vi "Set Arm State.vi"(8 "error in":errorcluster, 9 "PotDevRef":T12={"DevStatus"={"status"=FALSE, "code"=0, "source"=""}, "Controller"=enum."Controller 1", "Analog Channel"=enum."AI 2", "Invert Output"=FALSE}, 10 "MotorControlDevRef":T3={"DeviceStatus"={"status"=FALSE, "code"=0, "source"=""}, "Type"=enum."CANTalonSRX", "PWM"={"Controller"=enum."Controller 1", "PWM Channel"=enum."PWM 1", "DeadBand"={"Name"="", "maxPositivePwm"=0, "minPositivePwm"=0, "centerPwm"=0, "maxNegativePwm"=0, "minNegativePwm"=0, "angularRange"=0}}, "CAN"={"Device Number"=2, "Control Mode"=enum."Percent VBus", "Semaphore"=refnum, "Max Vout"=12.0, "TalonSRX Control Mode"=enum."Percent VBus"}, "Invert"=TRUE, "TransformRef"=refnum, "InvTransformRef"=refnum}, 11 "State":T2) -> (0 "error out":errorcluster, 1 "Good enough?":bool=TRUE)   [LabVIEW 2014]
doc: "Actuate the arm motors using a PID loop based on the next state."
uses:
  Arm State.ctl
  <vilib>/Rock Robotics/WPI/Potentiometer/WPI_PotentiometerDevRef.ctl
  <vilib>/Rock Robotics/SystemInterfaces/Typedef/FPGA_TypedefAnalogModule.ctl
  <vilib>/Rock Robotics/SystemInterfaces/AI/FPGA_AIChannel.ctl
  <vilib>/Rock Robotics/WPI/MotorControl/WPI_MotorControlDeviceRef.ctl
  <vilib>/Rock Robotics/WPI/MotorControl/WPI_MotorControlType.ctl
  <vilib>/Rock Robotics/SystemInterfaces/Typedef/FPGA_TypedefDigitalModule.ctl
  <vilib>/Rock Robotics/SystemInterfaces/DIO/FPGA_DIOPWMChannel.ctl
  <vilib>/Rock Robotics/WPI/PWM/WPI_PWMDeadband.ctl
  <vilib>/Rock Robotics/WPI/CAN/Jaguar/SubVIs/WPI_CANJaguar_ControlMode.ctl
  <vilib>/Rock Robotics/WPI/CAN/TalonSRX/WPI_CANTalonSRX_APIControlMode.ctl
  <vilib>/Rock Robotics/WPI/PWM/WPI_PWMTransform_ConPane.ctl
  Arm Angle Control Mode.ctl
  <vilib>/Rock Robotics/WPI/DriverStation/WPI_DriverStationRobotMode2.ctl
  <vilib>/Rock Robotics/Network Tables/SD Read Boolean.vi
  Robot Global Data.vi
  <vilib>/addons/control/pid/pid.llb/PID (DBL).vi
  <vilib>/Rock Robotics/Network Tables/SD Write Number.vi
  <vilib>/addons/control/pid/NI_PID_pid.lvlib
panel:
  in  "Tolerance":dbl=0.05 format="%#_13g"
  in  "PID?":bool=TRUE
  in  "Formula":i32=2
  in  "Tab Control":T1(tab)=enum."PID"
  in  "Vertical Setpoint":dbl=0.516 format="%#_13g"
  in  "output range":cluster{"output high":dbl, "output low":dbl}={"output high"=1.0, "output low"=-1.0}
  in  "PID gains":T15={"proportional gain (Kc)"=5.0, "integral time (Ti, min)"=0.0, "derivative time (Td, min)"=0.0} {"proportional gain (Kc)" min=0.0 max=1000.0 step=0.01; "integral time (Ti, min)" min=0.0 max=1000.0 step=0.0001; "derivative time (Td, min)" min=0.0 max=10000.0 step=0.001}
  in  "Lower Setpoint":dbl=0.088 format="%#_13g"
  in  "Raise Setpoint":dbl=0.252 format="%#_13g"
  in  "Level Setpoint":dbl=0.148 format="%#_13g"
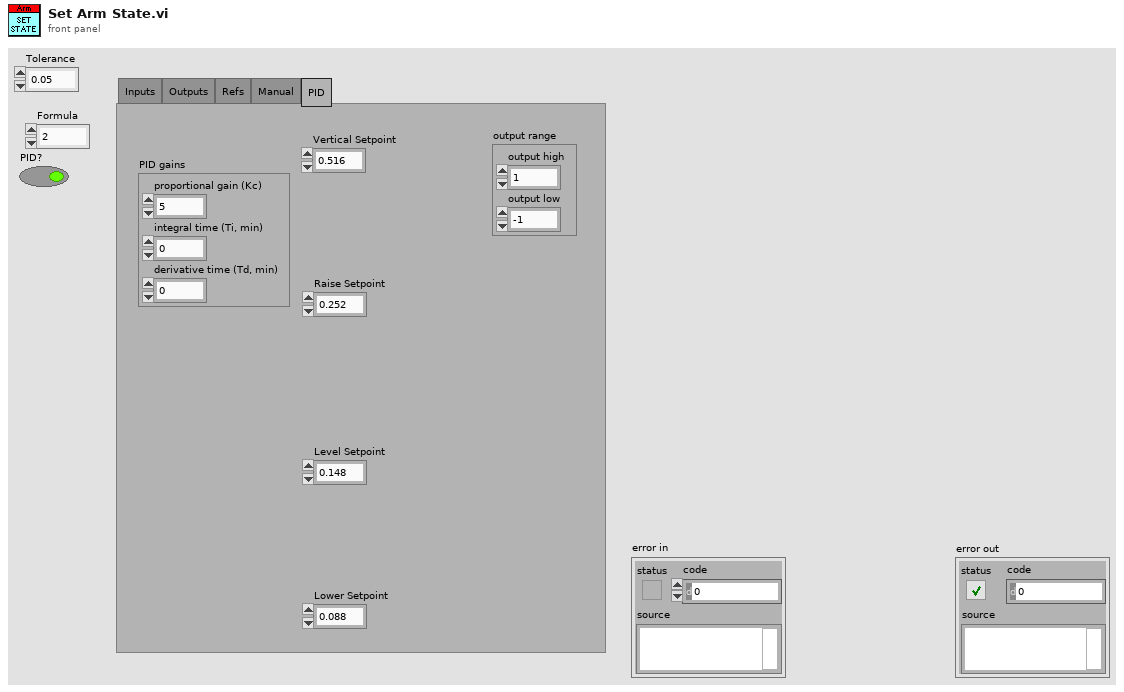
[diagram p1: front panel]
types:
  T1 = enum32{"Inputs", "Outputs", "Refs", "Manual", "PID"}
  T2 = typedef "Arm State.ctl" = enum16{"Ground", "Level", "Feeder", "Vertical"}
  T3 = typedef "WPI_MotorControlDeviceRef.ctl" = cluster{"DeviceStatus":errorcluster, "Type":T4, "PWM":cluster{"Controller":T5, "PWM Channel":T6, "DeadBand":T7}, "CAN":cluster{"Device Number":u8, "Control Mode":T8, "Semaphore":T9, "Max Vout":dbl, "TalonSRX Control Mode":T10}, "Invert":bool, "TransformRef":T11, "InvTransformRef":T11}
  T4 = typedef "WPI_MotorControlType.ctl" = enum16{"PWM", "CAN", "CANTalonSRX"}
  T5 = typedef "FPGA_TypedefDigitalModule.ctl" = enum16{"Controller 1"}
  T6 = typedef "FPGA_DIOPWMChannel.ctl" = enum8{"PWM 0", "PWM 1", "PWM 2", "PWM 3", "PWM 4", "PWM 5", "PWM 6", "PWM 7", "PWM 8", "PWM 9", "PWM MXP 0", "PWM MXP 1", "PWM MXP 2", "PWM MXP 3", "PWM MXP 4", "PWM MXP 5", "PWM MXP 6", "PWM MXP 7", "PWM MXP 8", "PWM MXP 9", "Invalid"}
  T7 = typedef "WPI_PWMDeadband.ctl" = cluster{"Name":string, "maxPositivePwm":i32, "minPositivePwm":i32, "centerPwm":i32, "maxNegativePwm":i32, "minNegativePwm":i32, "angularRange":u16}
  T8 = typedef "WPI_CANJaguar_ControlMode.ctl" = enum8{"Percent VBus", "Current", "Speed", "Position", "Voltage"}
  T9 = typedef "Semaphore RefNum" = refnum<k1>
  T10 = typedef "WPI_CANTalonSRX_APIControlMode.ctl" = enum8{"Percent VBus", "Speed", "Position", "Slave", "Unchanged / Invalid"}
  T11 = typedef "WPI_PWMTransform_ConPane.ctl" = refnum<vi>
  T12 = typedef "WPI_PotentiometerDevRef.ctl" = cluster{"DevStatus":errorcluster, "Controller":T13, "Analog Channel":T14, "Invert Output":bool}
  T13 = typedef "FPGA_TypedefAnalogModule.ctl" = enum16{"Controller 1"}
  T14 = typedef "FPGA_AIChannel.ctl" = enum8{"AI 0", "AI 1", "AI 2", "AI 3", "AI MXP 0", "AI MXP 1", "AI MXP 2", "AI MXP 3", "Invalid"}
  T15 = cluster{"proportional gain (Kc)":dbl, "integral time (Ti, min)":dbl, "derivative time (Td, min)":dbl}
  T16 = typedef "Arm Angle Control Mode.ctl" = enum16{"PID", "PID to Manual", "Manual"}
  T17 = typedef "WPI_DriverStationRobotMode2.ctl" = enum16{"Autonomous Disabled", "Autonomous Enabled", "Teleop Disabled", "Teleop Enabled", "Disconnected", "Finish", "Test Disabled", "Test Enabled", "Emergency Stopped"}
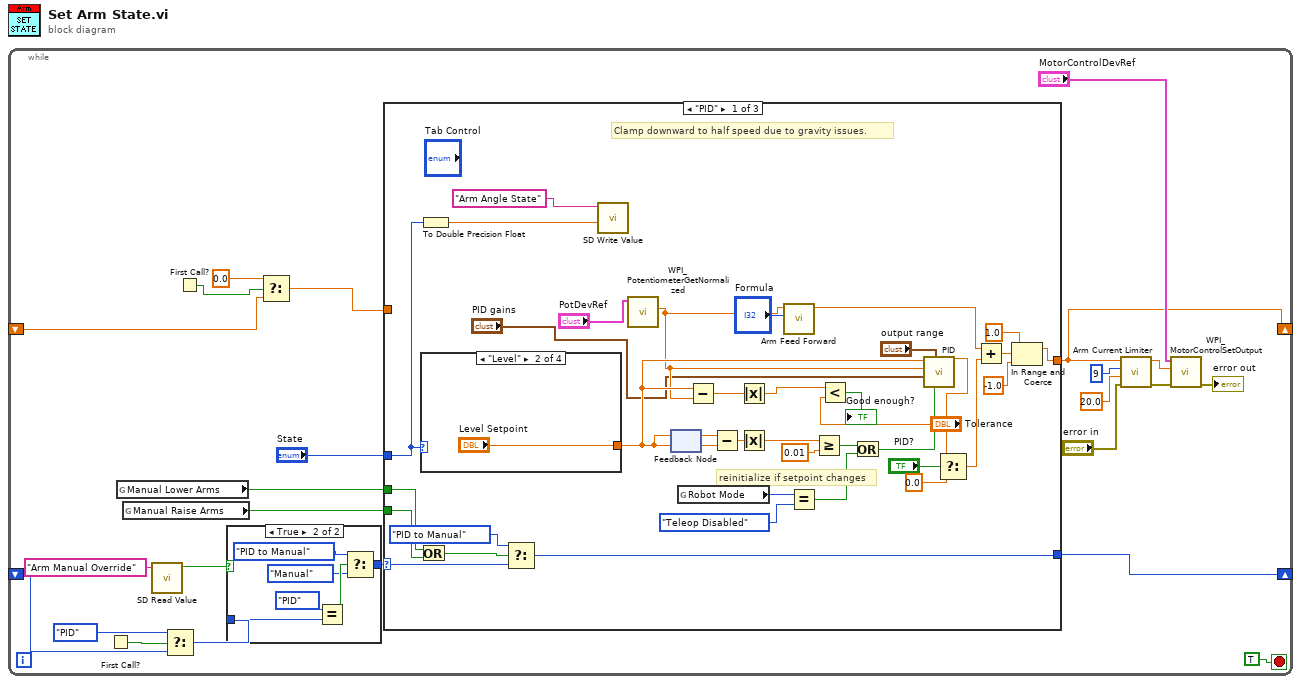
[diagram p0: block diagram]
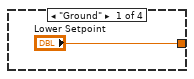
[diagram p3: hidden frame]
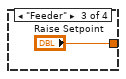
[diagram p4: hidden frame]
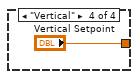
[diagram p5: hidden frame]
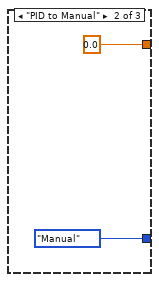
[diagram p6: hidden frame]
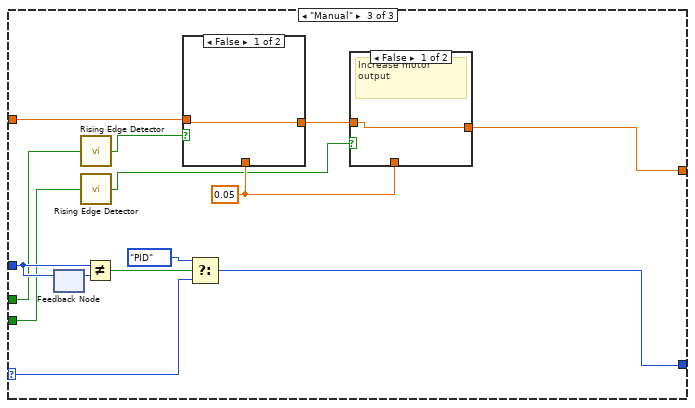
[diagram p7: hidden frame]
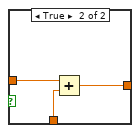
[diagram p8: hidden frame]
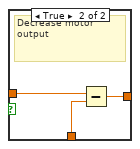
[diagram p9: hidden frame]
diagram:
  n1 = while {
    shift-right: [w23] -> _
    shift-left: _ -> [w18]
    shift-right: [w9] -> _
    shift-left: _ -> [w7]
    stop <- TRUE stop-if-true
    n2 = First Call?() -> (First Call?: T/F=w20:bool)
    n3 = global read "Robot Global Data.vi" "Manual Lower Arms"() -> (w22:bool)
    n4 = global read "Robot Global Data.vi" "Manual Raise Arms"() -> (w24:bool)
    n5 = call-poly <vilib>:"SD Read Value.vi"("Name"="Arm Manual Override") -> ("Boolean"=w3:bool)  [unwired: 8 in, 2 out]
    n6 = Select(t=Arm_Angle_Control_Mode."PID", s=w20, f=w18) -> (s? t:f=w2:T16)
    n7 = First Call?() -> (First Call?: T/F=w5:bool)
    n8 = case shown="True" w3 {
      tunnel: w2 -> [w25 w31]
      tunnel: [w25 w29] -> w1
      frame False {
      }
      frame True {
        n9 = Equal?(x=Arm_Angle_Control_Mode."PID", y=w31) -> (x = y?=w28:bool)
        n10 = Select(t=Arm_Angle_Control_Mode."PID to Manual", s=w28, f=Arm_Angle_Control_Mode."Manual") -> (s? t:f=w29:T16)
      }
    }
    n11 = Select(t=0.0, s=w5, f=w7) -> (s? t:f=w4:dbl)
    n12 = case shown="\"PID\"" w1 {
      selector: w1 -> [w65 _ w84]
      tunnel: "State" -> [w66 _ w85]
      tunnel: [w32 0.0 ("t") w80] -> w9
      tunnel: w22 -> [w67 _ w83]
      tunnel: w24 -> [w68 _ w82]
      tunnel: [w62 Arm_Angle_Control_Mode."Manual" w88] -> w23
      tunnel: w4 -> [_ _ w81]
      frame "PID" {
        # "Clamp downward to half speed due to gravity issues."
        # "reinitialize if setpoint changes"
        n13 = Or(x=w67, y=w68) -> (x .or. y?=w61:bool)
        n14 = To Double Precision Float(number=w66) -> (double precision float=w64:dbl)
        n15 = case shown="\"Level\"" w66 {
          tunnel: ["Lower Setpoint" "Level Setpoint" "Raise Setpoint" "Vertical Setpoint"] -> w45
          frame "Ground" {
          }
          frame "Level" {
          }
          frame "Feeder" {
          }
          frame "Vertical" {
          }
        }
        n16 = Select(t=Arm_Angle_Control_Mode."PID to Manual", s=w61, f=w65) -> (s? t:f=w62:T16)
        n17 = call-poly <vilib>:"SD Write Value.vi"("Numeric"=w64, "Name"="Arm Angle State") -> ()  [unwired: 8 in, 2 out]
        n18 = call <vilib>:"WPI_PotentiometerGetNormalized.vi"("PotDevRef"="PotDevRef") -> ("Normalized Value"=w43:dbl)  [unwired: 8 in, 2 out]
        n19 = feedback #1() -> (w44:dbl)  [unwired: 1 in]
        n20 = feedback-in #1(w45) -> ()
        n21 = global read "Robot Global Data.vi" "Robot Mode"() -> (w52:T17)
        n22 = Subtract(x=w45, y=w43) -> (x-y=w50:dbl)
        n23 = Subtract(x=w44, y=w45) -> (x-y=w56:dbl)
        n24 = Absolute Value(x=w50) -> (abs(x)=w49:dbl)
        n25 = Absolute Value(x=w56) -> (abs(x)=w57:dbl)
        n26 = call "Arm Feed Forward.vi"("Numeric"="Formula", "Arm Position"=w43) -> ("Feed Forward"=w42:dbl)  [unwired: 9 in]
        n27 = Equal?(x=w52, y=WPI_DriverStationRobotMode2."Teleop Disabled") -> (x = y?=w54:bool)
        n28 = Greater Or Equal?(x=w57, y=0.01) -> (x >= y?=w58:bool)
        n29 = Less?(x=w49, y="Tolerance") -> (x < y?=→"Good enough?":bool)
        n30 = Or(x=w58, y=w54) -> (x .or. y?=w59:bool)
        n31 = call-poly <vilib>:"PID.vi"("reinitialize? (F)"=w59, "output range"="output range", "PID gains"="PID gains", "process variable"=w43, "setpoint"=w45) -> ("output"=w39:dbl)  [unwired: 5 in, 1 out]
        n32 = Select(t=w39, s="PID?", f=0.0) -> (s? t:f=w38:dbl)
        n33 = Add(x=w42, y=w38) -> (x+y=w35:dbl)
        n34 = In Range and Coerce(upper limit=1.0, x=w35, lower limit=-1.0) -> (coerced(x)=w32:dbl)  [unwired: 1 out]
      }
      frame "PID to Manual" {
      }
      frame "Manual" {
        w77 = 0.05 ("y")
        n35 = feedback #2() -> (w86:T2)  [unwired: 1 in]
        n36 = feedback-in #2(w85) -> ()
        n37 = call "Rising Edge Detector.vi"("Input"=w83) -> ("Rising edge?"=w79:bool)
        n38 = call "Rising Edge Detector.vi"("Input"=w82) -> ("Rising edge?"=w76:bool)
        n39 = Not Equal?(x=w85, y=w86) -> (x != y?=w87:bool)
        n40 = case shown="False" w79 {
          tunnel: w81 -> [w93 w96]
          tunnel: [w93 w95] -> w78
          tunnel: w77 -> [_ w94]
          frame False {
          }
          frame True {
            # "Decrease motor output"
            n41 = Subtract(x=w96, y=w94) -> (x-y=w95:dbl)
          }
        }
        n42 = Select(t=Arm_Angle_Control_Mode."PID", s=w87, f=w84) -> (s? t:f=w88:T16)
        n43 = case shown="False" w76 {
          tunnel: w78 -> [w89 w92]
          tunnel: w77 -> [_ w91]
          tunnel: [w89 w90] -> w80
          frame False {
            # "Increase motor\noutput"
          }
          frame True {
            n44 = Add(x=w92, y=w91) -> (x+y=w90:dbl)
          }
        }
      }
    }
    n45 = call "Arm Current Limiter.vi"("Motor Input"=w9, "PDP Channel for arm motor"=9, "Max Current"=20.0, "error in"="error in") -> ("Set Motor To"=w17:dbl, "error out"=w16:errorcluster)  [unwired: 5 in]
    n46 = call <vilib>:"WPI_MotorControlSetOutput.vi"("error in (no error)"=w16, "Output"=w17, "MotorControlDevRef"="MotorControlDevRef") -> ("error out"=→"error out":errorcluster)  [unwired: 6 in, 2 out]
  }
